vi "mhk_data logger.vi"() -> ()   [LabVIEW 2010]
panel:
  out "2D Array":i32[][](array[numeric])
  out "Outer Loop \nCounter":i32
  out "array":i32[](array[numeric])
  out "Inner Loop Counter":i32
  in  "# of Columns":u8
  in  "# of Rows":u8
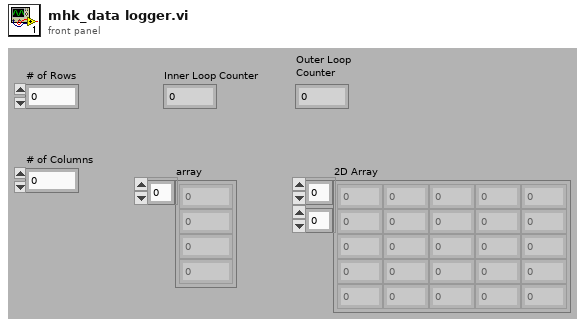
[diagram p1: front panel]
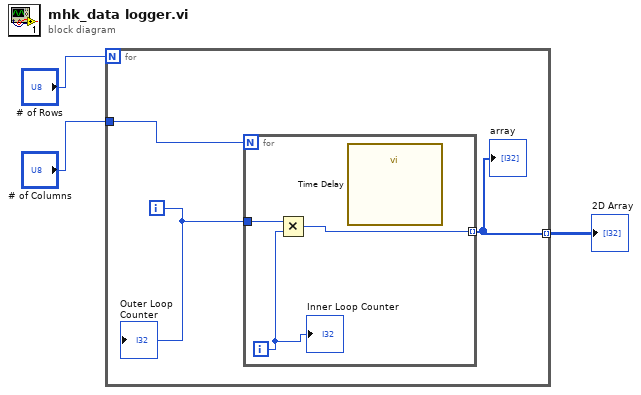
[diagram p0: block diagram]
diagram:
  n1 = for {
    N: "# of Rows" -> [_]
    tunnel: "# of Columns" -> [w4]
    tunnel: [w5] -> w1 mode=indexing
    i -> [w6]
    n2 = for {
      N: w4 -> [_]
      tunnel: w6 -> [w9]
      tunnel: [w7] -> w5 mode=indexing
      i -> [w8]
      n3 = Multiply(x=w9, y=w8) -> (x*y=w7:i32)
      n4 = call "Time Delay"() -> ()  [unwired: 11 in, 1 out]
      "Inner Loop Counter" <- w8
    }
    "array" <- w5
    "Outer Loop \nCounter" <- w6
  }
  "2D Array" <- w1
